vi "超标浓度设置.vi"(11 "输入":T2) -> (3 "输出":T1)   [LabVIEW 2016, in "德润DR803L超标留样.lvlib"]
uses:
  <vilib>/Utility/miscctls.llb/LVPointTypeDef.ctl
panel:
  in  "COD超标浓度":dbl
  in  "ORP超标浓度":dbl
  in  "蓝绿藻超标浓度":dbl
  in  "藻密度超标浓度":dbl
  in  "叶绿素a超标浓度":dbl
  in  "浊度超标浓度":dbl
  in  "电导率超标浓度":dbl
  in  "溶解氧超标浓度":dbl
  in  "PH超标浓度":dbl
  in  "取消":bool
  in  "确定":bool
  in  "CODCr超标浓度":dbl
  in  "CODMn超标浓度":dbl
  in  "总氮超标浓度":dbl
  in  "总磷超标浓度":dbl
  in  "氨氮超标浓度":dbl
  # "超标浓度报警配置"
  # "cells/mL"
  # "/"
  # "mg/L"
  # "cells/mL"
  # "mg/L"
  # "mg/L"
  # "/"
  # "μs/cm"
  # "mg/L"
  # "mg/L"
  # "NTU"
  # "mg/L"
  # "μg/L"
  # "mg/L"
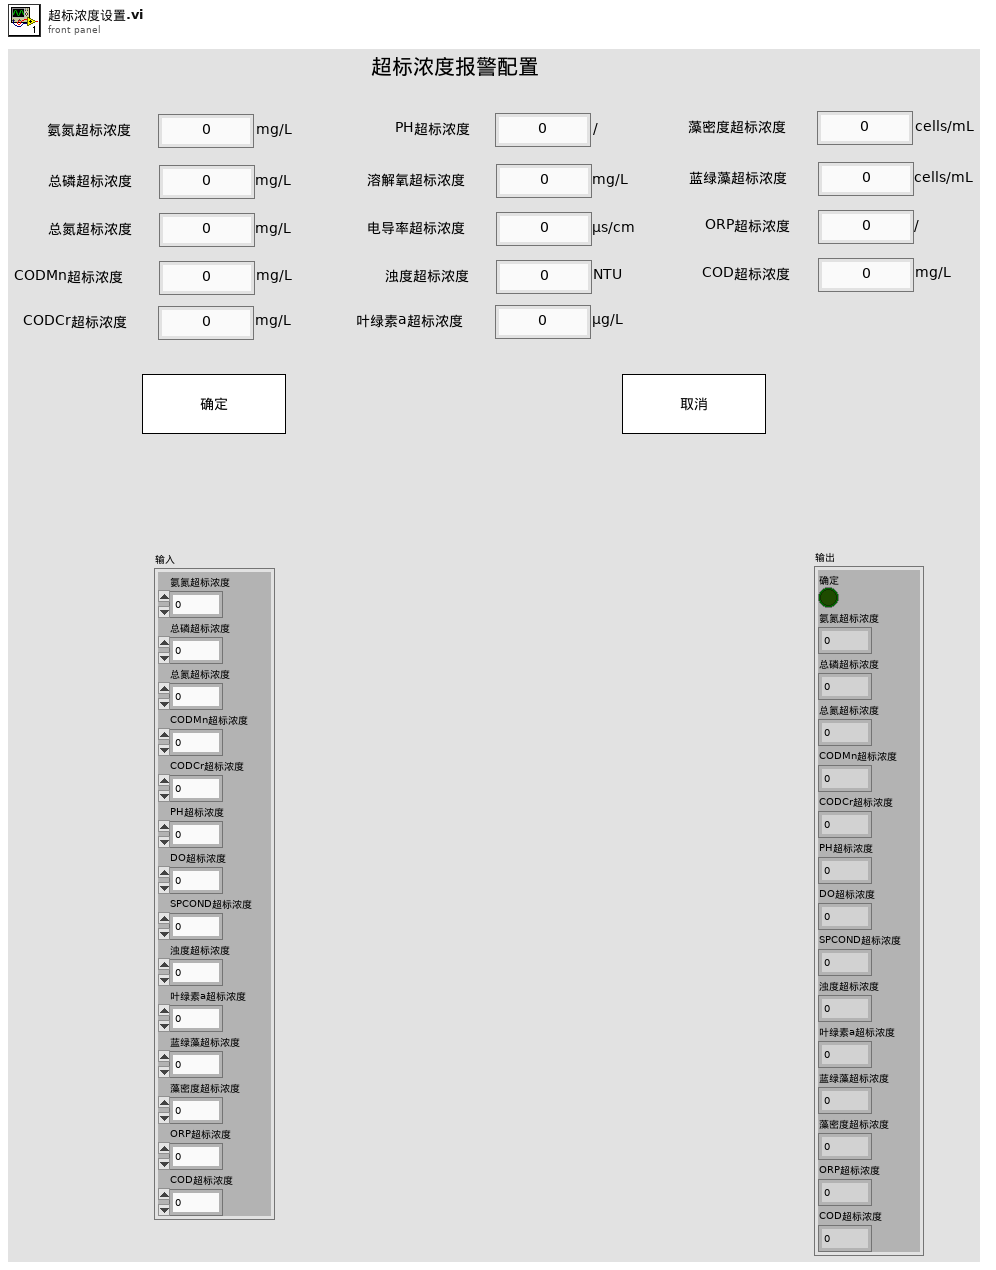
[diagram p1: front panel]
types:
  T1 = cluster{"确定":bool, "氨氮超标浓度":dbl, "总磷超标浓度":dbl, "总氮超标浓度":dbl, "CODMn超标浓度":dbl, "CODCr超标浓度":dbl, "PH超标浓度":dbl, "DO超标浓度":dbl, "SPCOND超标浓度":dbl, "浊度超标浓度":dbl, "叶绿素a超标浓度":dbl, "蓝绿藻超标浓度":dbl, "藻密度超标浓度":dbl, "ORP超标浓度":dbl, "COD超标浓度":dbl}
  T2 = cluster{"氨氮超标浓度":dbl, "总磷超标浓度":dbl, "总氮超标浓度":dbl, "CODMn超标浓度":dbl, "CODCr超标浓度":dbl, "PH超标浓度":dbl, "DO超标浓度":dbl, "SPCOND超标浓度":dbl, "浊度超标浓度":dbl, "叶绿素a超标浓度":dbl, "蓝绿藻超标浓度":dbl, "藻密度超标浓度":dbl, "ORP超标浓度":dbl, "COD超标浓度":dbl}
  T3 = typedef "LVPointTypeDef.ctl" = cluster{"Horizontal":i16, "Vertical":i16}
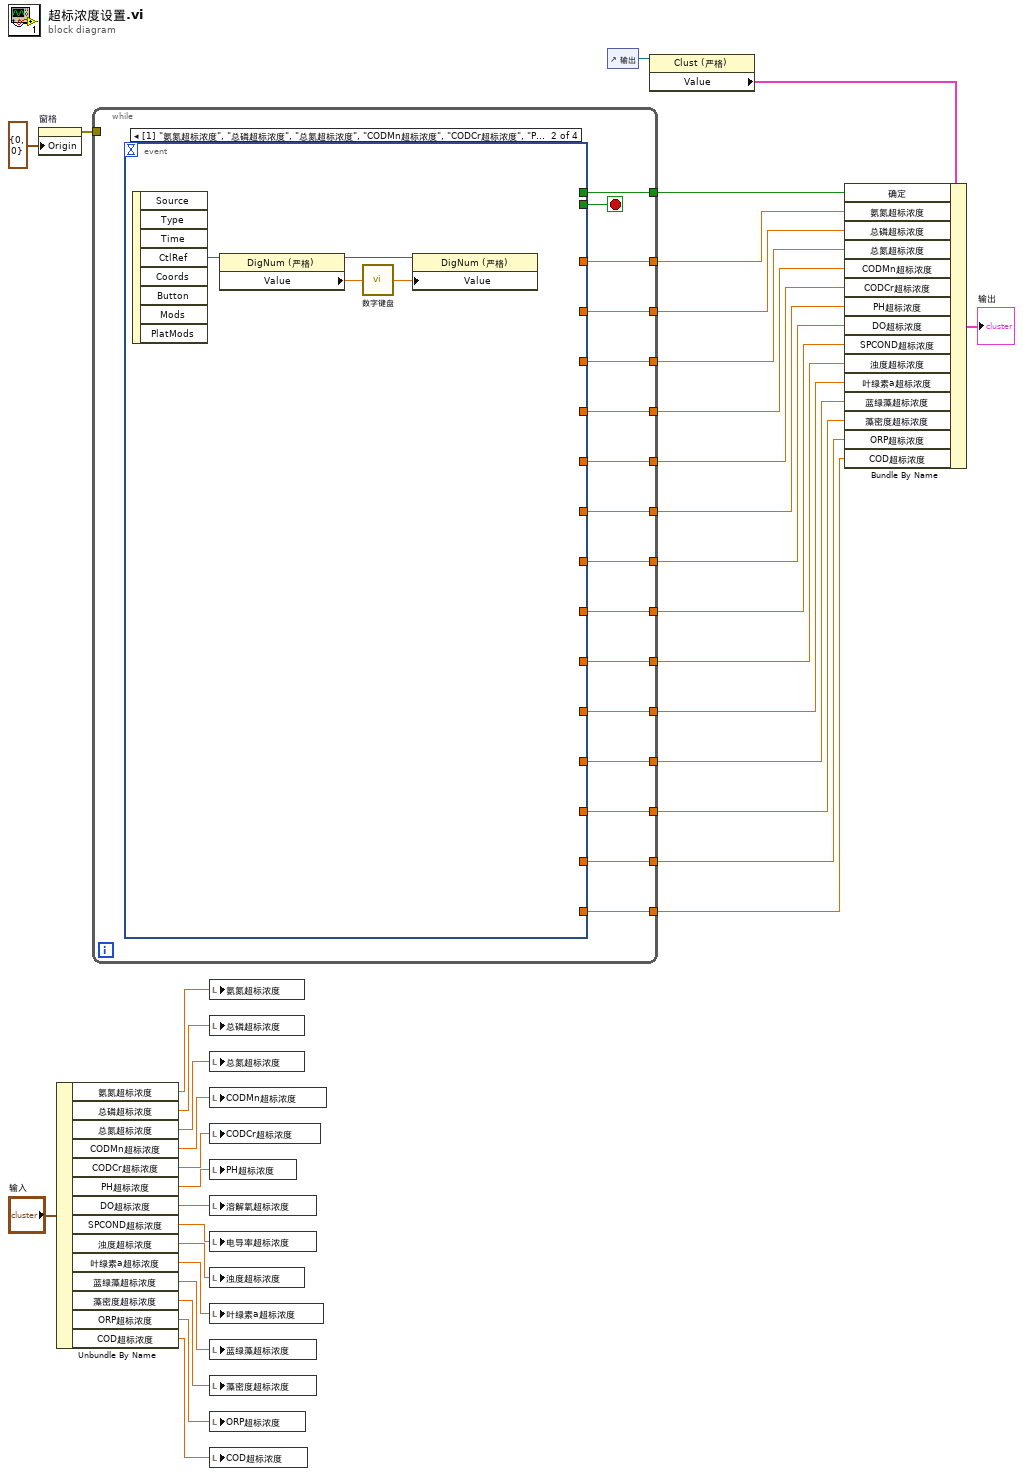
[diagram p0: block diagram]
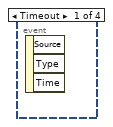
[diagram p2: hidden frame]
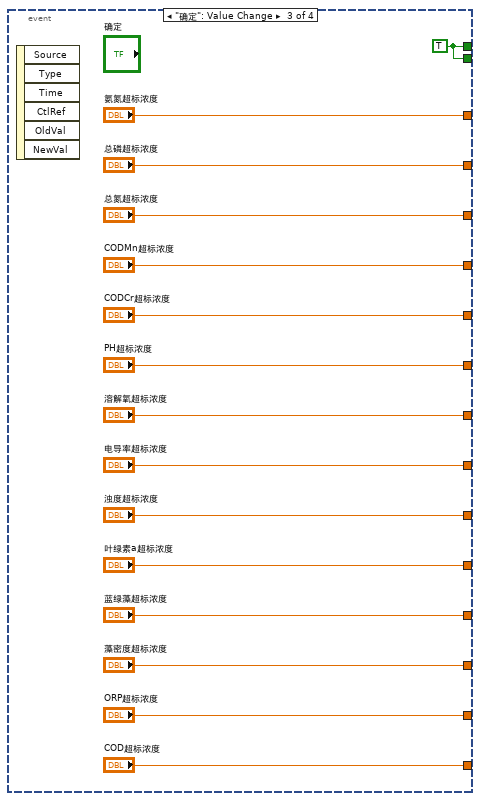
[diagram p3: hidden frame]
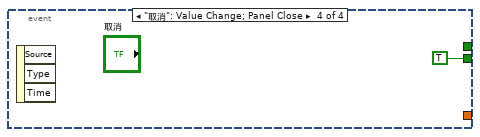
[diagram p4: hidden frame]
diagram:
  n1 = property on="窗格" class="Pane"("Origin"=T3 {"Horizontal"=0, "Vertical"=0} ("原点")) -> (error out=w10:errorcluster)  [unwired: 2 in, 1 out]
  n2 = Unbundle By Name("输入") -> ("氨氮超标浓度"=w27:dbl, "总磷超标浓度"=w26:dbl, "总氮超标浓度"=w25:dbl, "CODMn超标浓度"=w24:dbl, "CODCr超标浓度"=w23:dbl, "PH超标浓度"=w19:dbl, "DO超标浓度"=w18:dbl, "SPCOND超标浓度"=w17:dbl, "浊度超标浓度"=w16:dbl, "叶绿素a超标浓度"=w15:dbl, "蓝绿藻超标浓度"=w14:dbl, "藻密度超标浓度"=w13:dbl, "ORP超标浓度"=w12:dbl, "COD超标浓度"=w11:dbl)
  n3 = while {
    tunnel: [w50] -> w34
    tunnel: [w49] -> w33
    tunnel: [w48] -> w32
    tunnel: [w47] -> w31
    tunnel: [w46] -> w30
    tunnel: [w45] -> w29
    tunnel: w10 -> [_]
    tunnel: [w44] -> w9
    tunnel: [w43] -> w8
    tunnel: [w42] -> w7
    tunnel: [w41] -> w6
    tunnel: [w40] -> w5
    tunnel: [w39] -> w4
    tunnel: [w38] -> w3
    tunnel: [w37] -> w2
    tunnel: [w36] -> w1
    stop <- w51 stop-if-true
    n4 = event shown="[1] \"氨氮超标浓度\", \"总磷超标浓度\", \"总氮超标浓度\", \"CODMn超标浓度\", \"CODCr超标浓度\", \"PH超标浓度\", \"溶解氧超标浓度\", \"电导率超标浓度\", \"浊度超标浓度\", \"叶绿素a超标浓度\", \"藻密度超标浓度\", \"蓝绿藻超标浓度\", \"ORP超标浓度\", \"COD超标浓度\": 鼠标按下" {
      selector: _ -> [_ _ _ _]
      dyn-events: _ -> [_ _ _ _]
      timeout: _ -> [_ _ _ _]
      tunnel: [_ _ w70 TRUE] -> w51
      tunnel: [_ _ w70 _] -> w50
      tunnel: [_ _ "氨氮超标浓度" _] -> w49
      tunnel: [_ _ "总磷超标浓度" _] -> w48
      tunnel: [_ _ "总氮超标浓度" _] -> w47
      tunnel: [_ _ "CODMn超标浓度" _] -> w46
      tunnel: [_ _ "CODCr超标浓度" _] -> w45
      tunnel: [_ _ "PH超标浓度" _] -> w44
      tunnel: [_ _ "溶解氧超标浓度" _] -> w43
      tunnel: [_ _ "电导率超标浓度" _] -> w42
      tunnel: [_ _ "浊度超标浓度" _] -> w41
      tunnel: [_ _ "叶绿素a超标浓度" _] -> w40
      tunnel: [_ _ "蓝绿藻超标浓度" _] -> w39
      tunnel: [_ _ "藻密度超标浓度" _] -> w38
      tunnel: [_ _ "ORP超标浓度" _] -> w37
      tunnel: [_ _ "COD超标浓度" _] -> w36
      event Timeout {
        n5 = event-data() -> ()  [unwired: 1 in, 3 out]
      }
      event "氨氮超标浓度", "总磷超标浓度", "总氮超标浓度", "CODMn超标浓度", "CODCr超标浓度", "PH超标浓度", "溶解氧超标浓度", "电导率超标浓度", "浊度超标浓度", "叶绿素a超标浓度", "藻密度超标浓度", "蓝绿藻超标浓度", "ORP超标浓度", "COD超标浓度": Mouse Down {
        n6 = event-data() -> ("CtlRef"=w55:refnum<vi>)  [unwired: 1 in, 7 out]
        n7 = property class="DigNum (严格)"(reference=w55) -> (reference out=w53:refnum<vi>, "Value"=w54:dbl)  [unwired: 1 in, 1 out]
        n8 = call "数字键盘.vi"("OldNumber"=w54) -> ("NewNumber"=w52:sgl)
        n9 = property class="DigNum (严格)"(reference=w53, "Value"=w52) -> ()  [unwired: 1 in, 2 out]
      }
      event "确定": Value Change {
        w70 = TRUE
        n10 = event-data() -> ()  [unwired: 1 in, 6 out]
      }
      event "取消": Value Change; Panel Close {
        n11 = event-data() -> ()  [unwired: 1 in, 3 out]
      }
    }
  }
  n12 = local write "氨氮超标浓度"(w27) -> ()
  n13 = local write "总磷超标浓度"(w26) -> ()
  n14 = local write "总氮超标浓度"(w25) -> ()
  n15 = local write "CODMn超标浓度"(w24) -> ()
  n16 = local write "CODCr超标浓度"(w23) -> ()
  n17 = local write "PH超标浓度"(w19) -> ()
  n18 = local write "溶解氧超标浓度"(w18) -> ()
  n19 = local write "电导率超标浓度"(w17) -> ()
  n20 = local write "浊度超标浓度"(w16) -> ()
  n21 = local write "叶绿素a超标浓度"(w15) -> ()
  n22 = local write "蓝绿藻超标浓度"(w14) -> ()
  n23 = local write "藻密度超标浓度"(w13) -> ()
  n24 = local write "ORP超标浓度"(w12) -> ()
  n25 = local write "COD超标浓度"(w11) -> ()
  n26 = control-ref of="输出"() -> (w20:refnum<vi>)
  n27 = property class="Clust (严格)"(reference=w20) -> ("Value"=w35:T1)  [unwired: 1 in, 2 out]
  n28 = Bundle By Name(cluster=w35, "确定"=w34, "氨氮超标浓度"=w33, "总磷超标浓度"=w32, "总氮超标浓度"=w31, "CODMn超标浓度"=w30, "CODCr超标浓度"=w29, "PH超标浓度"=w9, "DO超标浓度"=w8, "SPCOND超标浓度"=w7, "浊度超标浓度"=w6, "叶绿素a超标浓度"=w5, "蓝绿藻超标浓度"=w4, "藻密度超标浓度"=w3, "ORP超标浓度"=w2, "COD超标浓度"=w1) -> (→"输出":T1)
